vi "CombineInterfacesMethod.vi"(8 "Error In":errorcluster, 11 "MulitInterface In":refnum<class "MulitInterface.lvclass">) -> (0 "Error Out":errorcluster, 3 "MulitInterface Out":refnum<class "MulitInterface.lvclass">)   [LabVIEW 2021, in "MulitInterface.lvclass"]
doc: "Example of inhertinace from 2 interfaces and use them methods."
uses:
  MulitInterface.lvclass
  Debug/Debug.lvclass
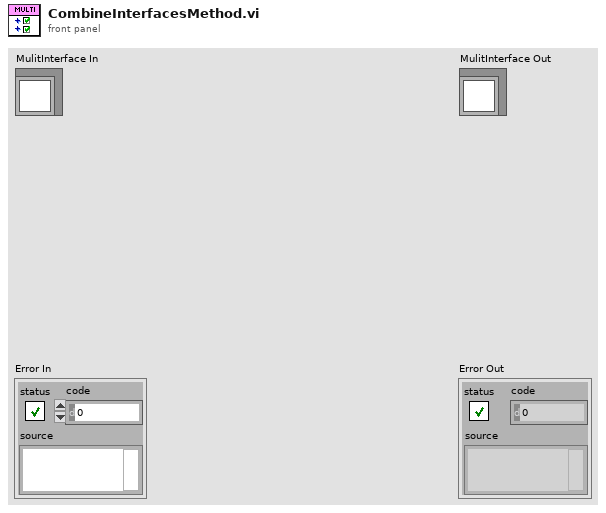
[diagram p1: front panel]
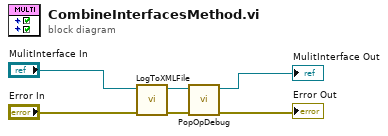
[diagram p0: block diagram]
diagram:
  n1 = call-dynamic "LogToXMLFile.vi"("Error In"="Error In", "LogClassData In"="MulitInterface In") -> ("Error Out"=w1:errorcluster, "LogClassData Out"=w6:refnum<class "MulitInterface.lvclass">)  [unwired: 8 in]
  n2 = call "PopOpDebug.vi"("Error In"=w1, "Debug in"=w6) -> ("Error Out"=→"Error Out":errorcluster, "Debug out"=→"MulitInterface Out":refnum<class "MulitInterface.lvclass">)  [unwired: 8 in]
